vi "Arduino_Communication.vi"() -> ()   [LabVIEW 2019]
uses:
  <vilib>/Instr/_visa.llb/VISA Configure Serial Port (Instr).vi
panel:
  in  "Read Position":bool
  out "Current Position":string
  in  "Full Cycle":bool
  in  "Baud rate (9600)":u32
  in  "VISA resource name":refnum<visa-resource-name>
  in  "Forward":bool
  in  "Stop":bool
  in  "Back":bool
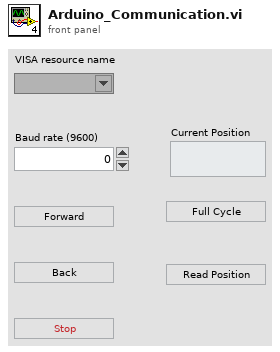
[diagram p1: front panel]
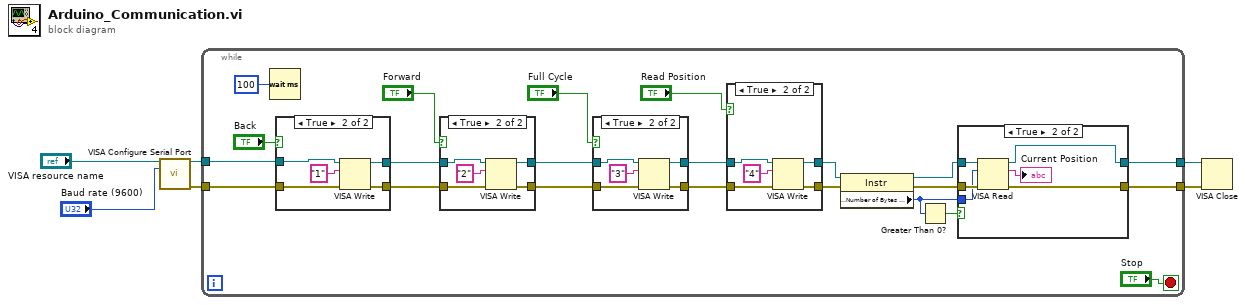
[diagram p0: block diagram]
diagram:
  n1 = call-poly "VISA Configure Serial Port"("VISA resource name"="VISA resource name", "baud rate (9600)"="Baud rate (9600)") -> ("VISA resource name out"=w6:refnum<visa-resource-name>, "error out"=w4:errorcluster)  [unwired: 12 in]
  n2 = while {
    tunnel: w6 -> [w28]
    tunnel: [w26] -> w5
    tunnel: w4 -> [w25]
    tunnel: [w23] -> w3
    stop <- "Stop" stop-if-true
    n3 = Wait (ms)(milliseconds to wait=u32 100) -> ()  [unwired: 1 out]
    n4 = case shown="True" "Back" {
      tunnel: w28 -> [w52 w57]
      tunnel: [w52 w56] -> w27
      tunnel: w25 -> [w51 w55]
      tunnel: [w51 w54] -> w24
      frame False {
      }
      frame True {
        n5 = VISA Write(VISA resource name=w57, write buffer="1", error in (no error)=w55) -> (VISA resource name out=w56:refnum<visa-resource-name>, error out=w54:errorcluster)  [unwired: 1 out]
      }
    }
    n6 = case shown="True" "Forward" {
      tunnel: w27 -> [w59 w64]
      tunnel: [w59 w63] -> w14
      tunnel: w24 -> [w58 w62]
      tunnel: [w58 w61] -> w13
      frame False {
      }
      frame True {
        n7 = VISA Write(VISA resource name=w64, write buffer="2", error in (no error)=w62) -> (VISA resource name out=w63:refnum<visa-resource-name>, error out=w61:errorcluster)  [unwired: 1 out]
      }
    }
    n8 = case shown="True" "Full Cycle" {
      tunnel: w14 -> [w37 w42]
      tunnel: [w37 w41] -> w10
      tunnel: w13 -> [w36 w40]
      tunnel: [w36 w39] -> w9
      frame False {
      }
      frame True {
        n9 = VISA Write(VISA resource name=w42, write buffer="3", error in (no error)=w40) -> (VISA resource name out=w41:refnum<visa-resource-name>, error out=w39:errorcluster)  [unwired: 1 out]
      }
    }
    n10 = case shown="True" "Read Position" {
      tunnel: w10 -> [w30 w35]
      tunnel: [w30 w34] -> w8
      tunnel: w9 -> [w29 w33]
      tunnel: [w29 w32] -> w7
      frame False {
      }
      frame True {
        n11 = VISA Write(VISA resource name=w35, write buffer="4", error in (no error)=w33) -> (VISA resource name out=w34:refnum<visa-resource-name>, error out=w32:errorcluster)  [unwired: 1 out]
      }
    }
    n12 = property class="Instr"(reference=w8, error in=w7) -> (reference out=w22:refnum<visa-resource-name>, error out=w21:errorcluster, "Serial Settings:Number of Bytes at Serial Port"=w19:u32)
    n13 = Greater Than 0?(x=w19) -> (x > 0?=w20:bool)
    n14 = case shown="True" w20 {
      tunnel: w22 -> [w44 w50]
      tunnel: [w44 w49] -> w26
      tunnel: w21 -> [w43 w48]
      tunnel: [w43 w47] -> w23
      tunnel: w19 -> [_ w46]
      frame False {
      }
      frame True {
        n15 = VISA Read(VISA resource name=w50, byte count=w46, error in (no error)=w48) -> (VISA resource name out=w49:refnum<visa-resource-name>, read buffer=→"Current Position":string, error out=w47:errorcluster)  [unwired: 1 out]
      }
    }
  }
  n16 = VISA Close(VISA resource name=w5, error in (no error)=w3) -> ()  [unwired: 1 out]
